vi "iv-sweep.vi"() -> ()   [LabVIEW 2010]
uses:
  <instrlib>/Keithley 24XX/Public/Data/Read (Multiple Points).vi
  <vilib>/Utility/file.llb/Write To Spreadsheet File (DBL).vi
  C/Program Files/National Instruments/LabVIEW 2016/instr.lib/Stanford Research 830/Stanford Research 830.lvlib
  C/Program Files/National Instruments/LabVIEW 2016/instr.lib/Keithley 2450/Keithley 2450.lvlib
  <instrlib>/Keithley 24XX/Keithley 24XX.lvlib
  <vilib>/Analysis/NI_AALBase.lvlib
panel:
  out "XY Graph 3":cluster{dbl[], dbl[]}(graph)={[], [3.246237e-08, 3.246237e-08]}
  in  "Parameter2 (1: X)  3":u16(ring)=2 items=["X"=1, "Y"=2, "R"=3, "Theta"=4, "Channel 1"=5, "Channel 2"=6, "Aux In 1"=7, "Aux In 2"=8, "Aux In 3"=9, "Aux In 4"=10]
  in  "Parameter (1: X) 3":u16(ring)=1 items=["X"=1, "Y"=2, "R"=3, "Theta"=4, "Channel 1"=5, "Channel 2"=6, "Aux In 1"=7, "Aux In 2"=8, "Aux In 3"=9, "Aux In 4"=10]
  in  "data number":dbl=100.0
  in  "offset(V)":dbl
  in  "Parameter2 (1: X)  2":u16(ring)=4 items=["X"=1, "Y"=2, "R"=3, "Theta"=4, "Channel 1"=5, "Channel 2"=6, "Aux In 1"=7, "Aux In 2"=8, "Aux In 3"=9, "Aux In 4"=10]
  out "PHASE":dbl=159.294
  out "LOCKIN2\n-THETA":cluster{dbl[], dbl[]}(graph)={[0.0005, 0.00045000000000000004, 0.0004, 0.00035, 0.00030000000000000003, 0.00025, 0.0002, 0.00015000000000000001, 0.0001, 5e-05, 0.0, 0.00024000000000000003, 0.00023, 0.00022, 0.00021, 0.0002, 0.00019, 0.00018, 0.00017, 0.00016, 0.00015000000000000001, 0.00014000000000000001, 0.00013000000000000002, 0.00012000000000000002, 0.00011, 0.0001, 9e-05, 8e-05, 7.000000000000001e-05, 6.000000000000001e-05, 5e-05, 4e-05, 3.0000000000000004e-05, 2e-05, 1e-05, 0.0], [159.294, 135.0, -5.628, -140.196, 157.518, -86.604, -109.212, 136.824, 42.054, -163.194, -5.196, -125.64, -38.532, -101.658, -53.202, 19.062, 69.636, -47.118, 180.0, -61.17, -36.72, 100.386, -110.046, -161.832, 112.836, 52.062, 88.626, -145.602, -128.772, -5.892, 43.392, 156.552, 66.102, -148.23, -19.77, -42.372]}
  in  "Parameter (1: X) 2":u16(ring)=3 items=["X"=1, "Y"=2, "R"=3, "Theta"=4, "Channel 1"=5, "Channel 2"=6, "Aux In 1"=7, "Aux In 2"=8, "Aux In 3"=9, "Aux In 4"=10]
  out "R Measurement 2":dbl=5.27132e-07
  out "LOVK2-r":cluster{dbl[], dbl[]}(graph)={[0.0005, 0.00045000000000000004, 0.0004, 0.00035, 0.00030000000000000003, 0.00025, 0.0002, 0.00015000000000000001, 0.0001, 5e-05, 0.0, 0.00024000000000000003, 0.00023, 0.00022, 0.00021, 0.0002, 0.00019, 0.00018, 0.00017, 0.00016, 0.00015000000000000001, 0.00014000000000000001, 0.00013000000000000002, 0.00012000000000000002, 0.00011, 0.0001, 9e-05, 8e-05, 7.000000000000001e-05, 6.000000000000001e-05, 5e-05, 4e-05, 3.0000000000000004e-05, 2e-05, 1e-05, 0.0], [5.27132e-07, 4.22822e-07, 3.52042e-07, 3.9302e-07, 4.33998e-07, 3.81844e-07, 5.01055e-07, 3.27827e-07, 2.14205e-07, 1.4715e-07, 1.84403e-07, 1.06171e-07, 5.92325e-07, 4.89879e-07, 2.83124e-07, 3.12926e-07, 2.19793e-07, 4.09784e-08, 4.65664e-08, 2.34694e-07, 3.63218e-07, 4.30273e-07, 2.58909e-07, 4.5635e-07, 7.11534e-07, 4.15372e-07, 6.98496e-07, 4.78703e-07, 5.42033e-07, 5.69973e-07, 2.6636e-07, 3.12926e-07, 2.88712e-07, 4.43311e-07, 2.62635e-07, 5.21544e-07]}
  in  "Clear Plot 2":bool
  in  "TRIGGER (1:EXTERNAL)":i32=1
  in  "REFERENCE(0:EXTERNAL)":i32
  in  "auto phase 2":bool=TRUE
  in  "manual phase 2":dbl
  in  "harm#2 2":dbl=1.0
  in  "Sine Output Amplitude (1 V) 3":dbl=0.05
  in  "Input Connection (0: Single-Ended Voltage)  2":u16(ring)=1 items=["Single-Ended Voltage", "Differential Voltage", "1 MOhm Current Gain", "100 MOhm Current Gain"]
  in  "frequency 2":dbl=50.0 format="%#_13g"
  in  "lockin-NL":refnum<visa-resource-name>="GPIB0::10::INSTR"
  out "XY Graph 2":cluster{dbl[], dbl[]}(graph)={[0.0005, 0.00045000000000000004, 0.0004, 0.00035, 0.00030000000000000003, 0.00025, 0.0002, 0.00015000000000000001, 0.0001, 5e-05, 0.0, 0.00025, 0.00024000000000000003, 0.00023, 0.00022, 0.00021, 0.0002, 0.00019, 0.00018, 0.00017, 0.00016, 0.00015000000000000001, 0.00014000000000000001, 0.00013000000000000002, 0.00012000000000000002, 0.00011, 0.0001, 9e-05, 8e-05, 7.000000000000001e-05, 6.000000000000001e-05, 5e-05, 4e-05, 3.0000000000000004e-05, 2e-05, 1e-05, 0.0], [8.888416918811881e-08, -1.8290904643564357e-07, 1.7707216663366337e-07, -2.2476362376237624e-08, 2.3799105722772277e-07, -3.8458769504950495e-08, -7.441385495049504e-09, -1.0435934356435644e-08, -1.0435934356435644e-08]}
  out "para2 Measurement":dbl=8.888416918811881e-08
  in  "auto phase":bool
  in  "manual phase":dbl
  in  "harm#2":dbl=2.0
  out "top gate leaking":dbl=-4.5445435609137164e-11
  out "top gate voltage":dbl format="%#_13g"
  in  "Compliance  Level (1uA)":dbl=3e-09
  in  "Source Mode  (0: Voltage)":u16(ring) items=["Voltage", "Current"]
  in  "top gate thickness":dbl=1.0
  in  "bottom gate thickness":dbl=1.0
  in  "pure field (T)/pure doping (F)":bool
  in  "Serial Configuration":T1={"Baud Rate"=9600, "Parity"=0, "Data Bits"=8, "Stop Bits"=10, "Flow Control"=0} {"Flow Control" items=["None", "XON/XOFF", "RTS/CTS", "XON/XOFF & RTS/CTS", "DTR/DSR", "XON/XOFF & DTR/DSR"]; "Stop Bits" items=["1.0"=10, "1.5"=15, "2.0"=20]; "Data Bits" items=["7"=7, "8"=8]; "Parity" items=["None", "Odd", "Even", "Mark", "Space"]; "Baud Rate" items=["300"=300, "600"=600, "1200"=1200, "2400"=2400, "4800"=4800, "9600"=9600, "19200"=19200]}
  in  "top gate address":refnum<visa-resource-name>="GPIB0::25::INSTR"
  out "loop run":i32=1
  in  "loop #":i32=1
  in  "Save data or not":bool
  in  "path (folder + filename)":string="C:\\Users\\User\\Data\\Jason\\07022019\\rl real other is ll\\pureE\\9v-100mv-avg-Pure E_100_new"
  in  "Clear Plot":bool
  out "XY Graph":cluster{dbl[], dbl[]}(graph)={[0.0005, 0.00045000000000000004, 0.0004, 0.00035, 0.00030000000000000003, 0.00025, 0.0002, 0.00015000000000000001, 0.0001, 5e-05, 0.0, 0.00025, 0.00024000000000000003, 0.00023, 0.00022, 0.00021, 0.0002, 0.00019, 0.00018, 0.00017, 0.00016, 0.00015000000000000001, 0.00014000000000000001, 0.00013000000000000002, 0.00012000000000000002, 0.00011, 0.0001, 9e-05, 8e-05, 7.000000000000001e-05, 6.000000000000001e-05, 5e-05, 4e-05, 3.0000000000000004e-05, 2e-05, 1e-05, 0.0], [8.142211237623763e-09, -5.9199106930693075e-09, 5.3011833564356435e-08, -6.179726722772277e-08, -1.642294698811881e-07, -1.2808030811881188e-08, -1.934349495049505e-08, 3.920102207920792e-08, 3.920102207920792e-08]}
  out "para1 Measurement":dbl=8.142211237623763e-09
  out "gate voltage":dbl format="%#_13g"
  out "gate leaking":string="3.246237E-08\n"
  in  "GATE STEP(uv)":i32=50
  in  "GATE Low Value (default 0)":dbl
  in  "GATE High Value":dbl=0.002
  in  "Function (0: Volts) 2":u16(ring) items=["Volts", "Current", "Resistance"]
  in  "Source Compaliance":dbl=3e-06
  in  "back gate address":refnum<visa-resource-name>="GPIB0::18::INSTR"
  in  "SD stabilization(S) 2":dbl=0.1 format="%#_13g"
  in  "Sine Output Amplitude (1 V) 2":dbl=2.0
  in  "LOCKIN-WAIT":dbl=0.5 format="%#_13g"
  in  "frequency":dbl=50.0 format="%#_13g"
  in  "Input Connection (0: Single-Ended Voltage)":u16(ring)=1 items=["Single-Ended Voltage", "Differential Voltage", "1 MOhm Current Gain", "100 MOhm Current Gain"]
  in  "LOCKIN address":refnum<visa-resource-name>="GPIB0::8::INSTR"
  # "Lock-in"
  # "top Gate Setting"
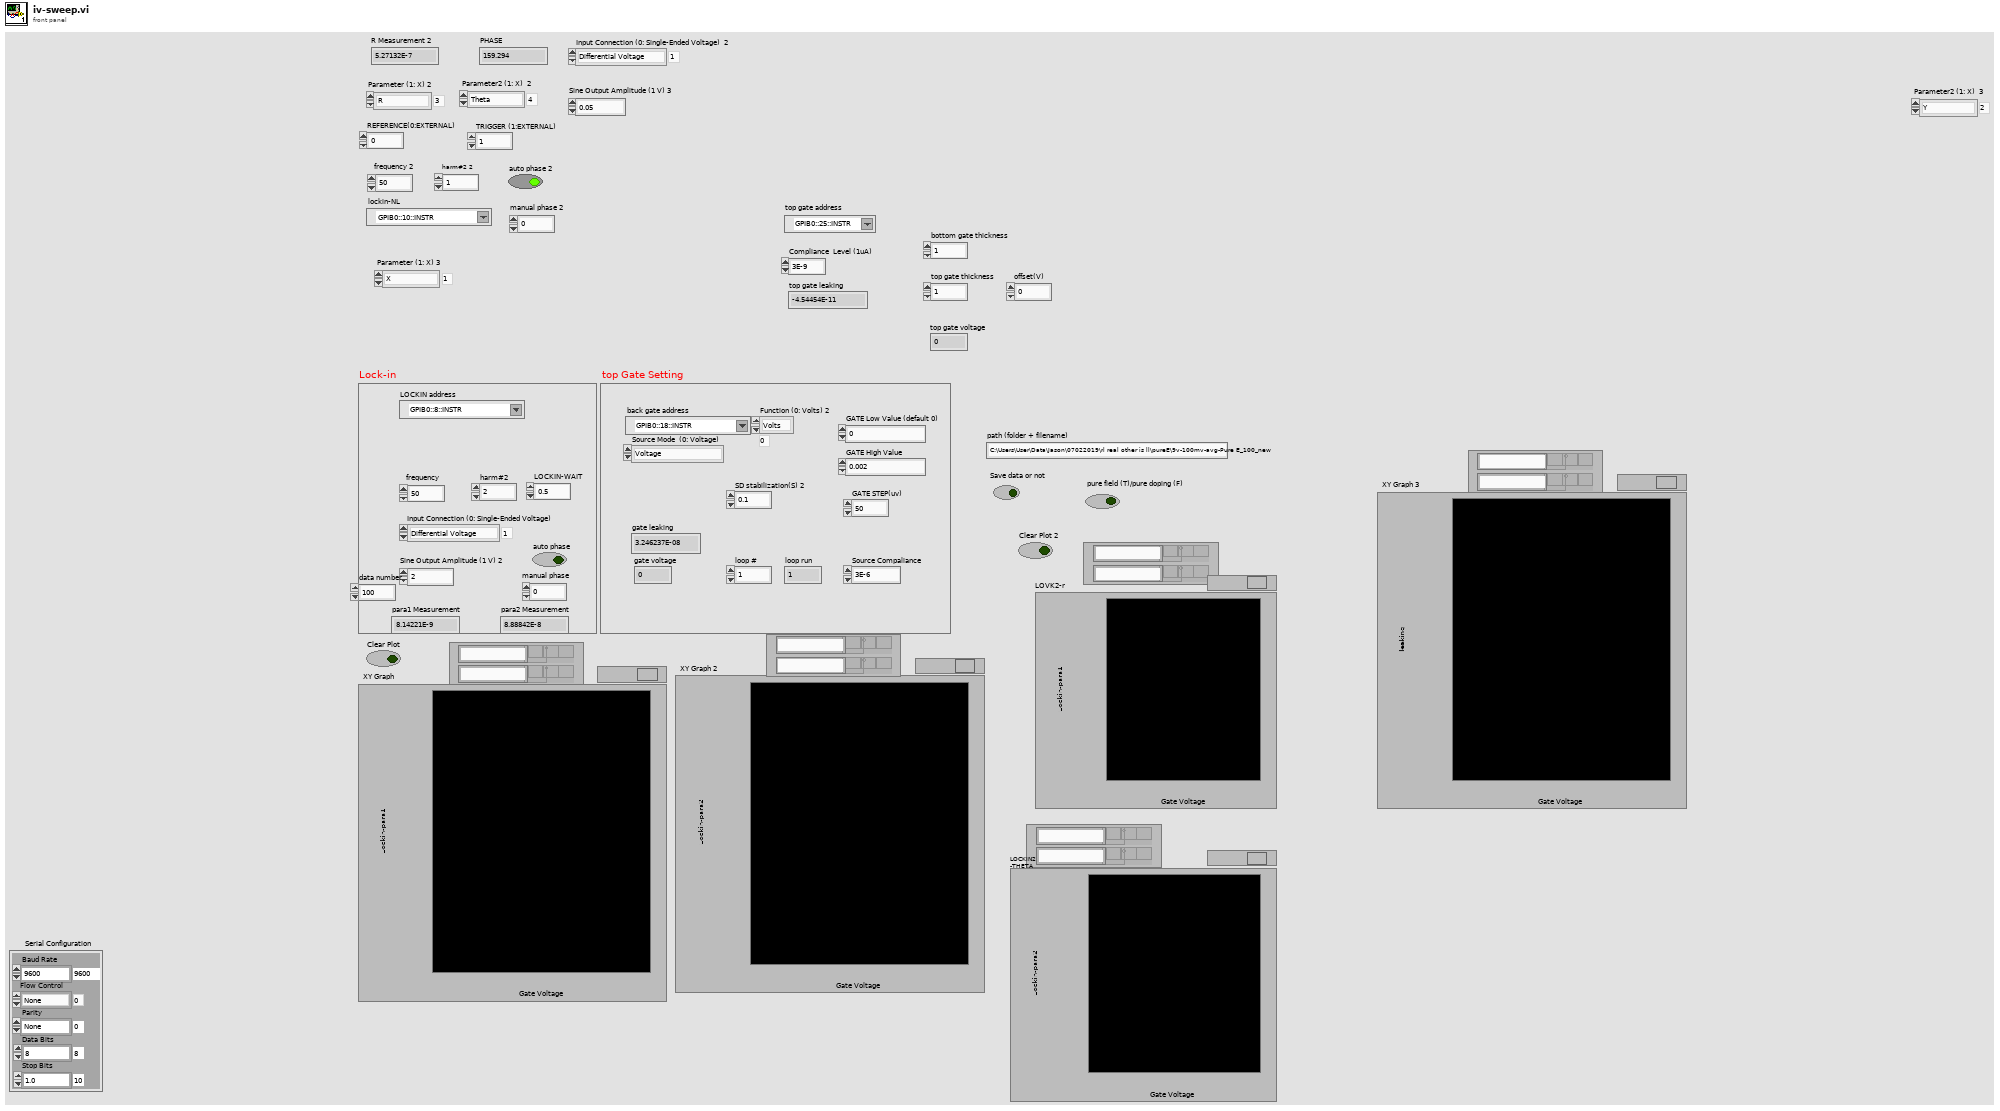
[diagram p1: front panel]
types:
  T1 = cluster{"Baud Rate":u32, "Parity":u16, "Data Bits":u16, "Stop Bits":u16, "Flow Control":u16}
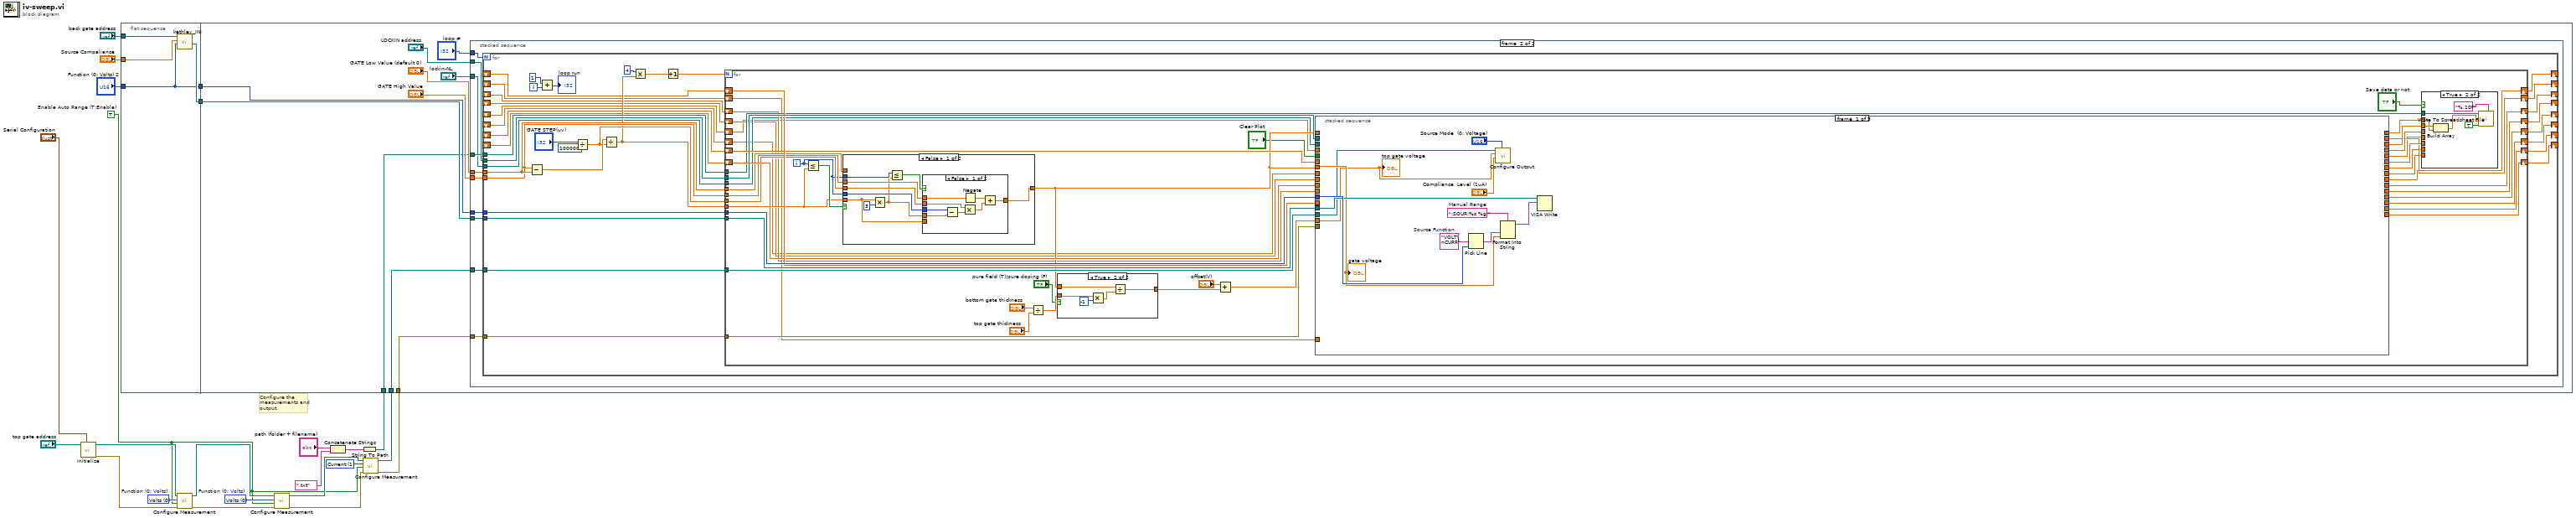
[diagram p0: block diagram]
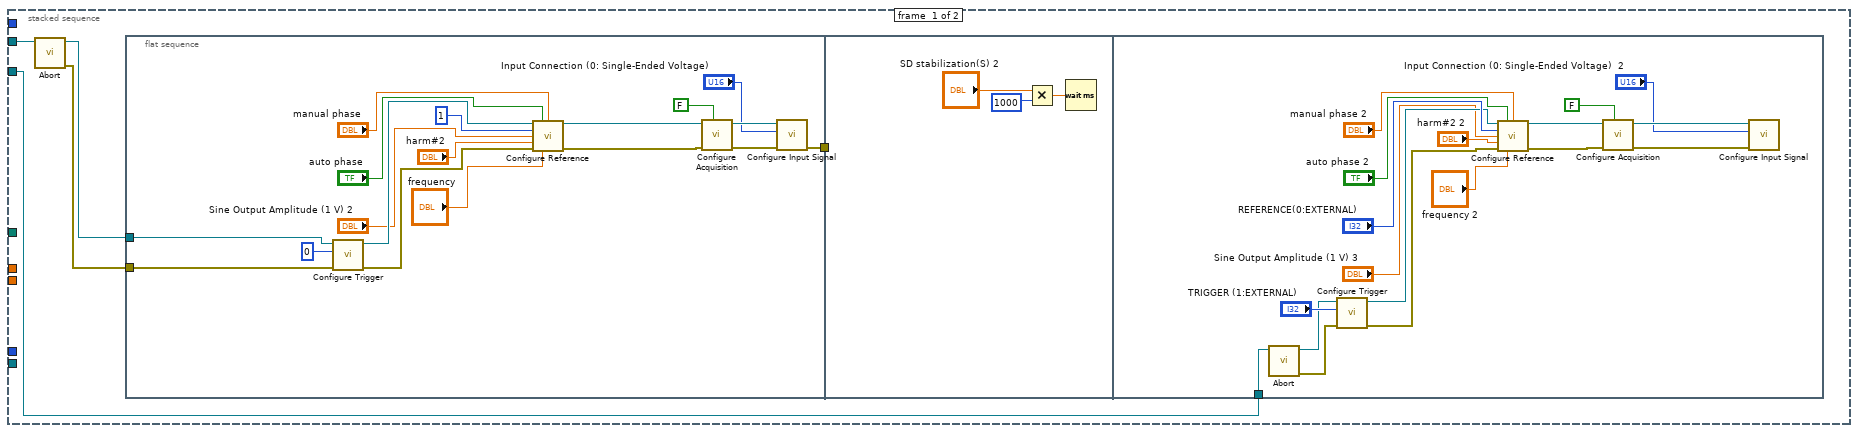
[diagram p2: hidden frame]
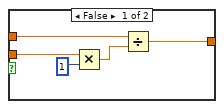
[diagram p3: hidden frame]
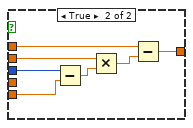
[diagram p5: hidden frame]
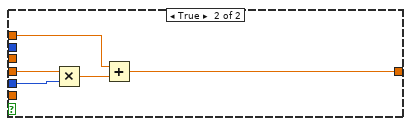
[diagram p6: hidden frame]
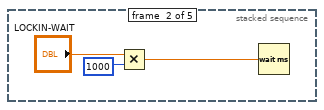
[diagram p7: hidden frame]
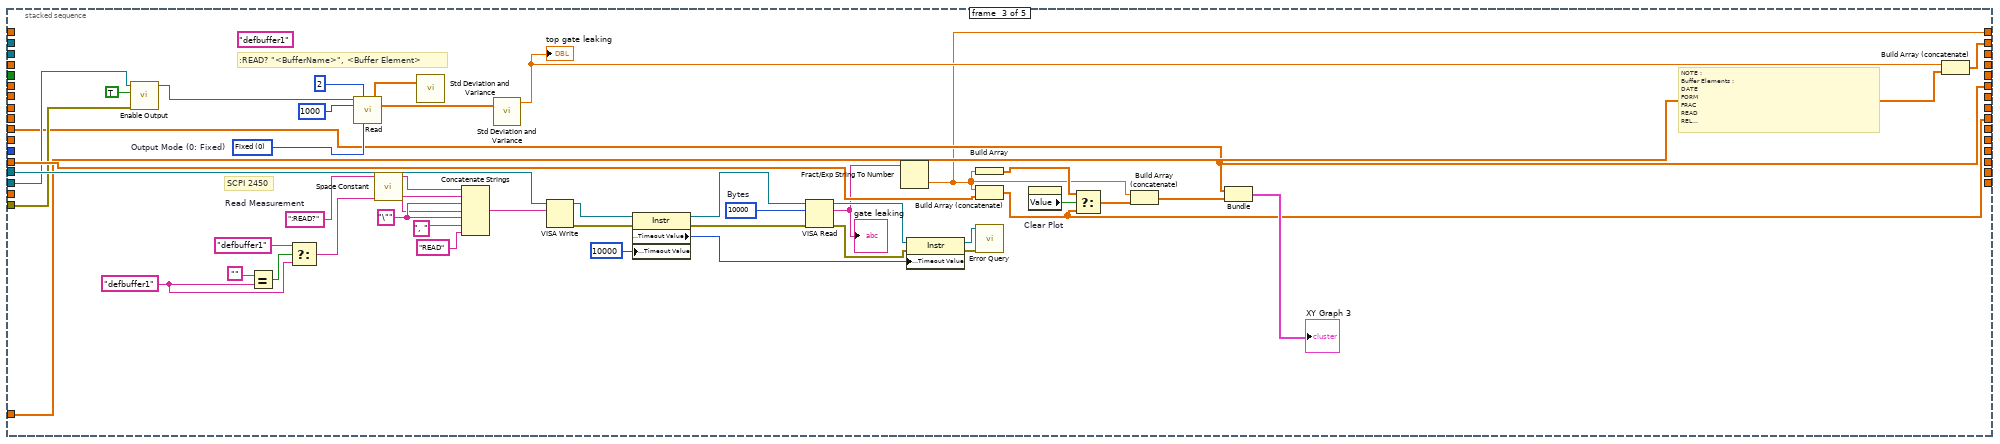
[diagram p8: hidden frame]
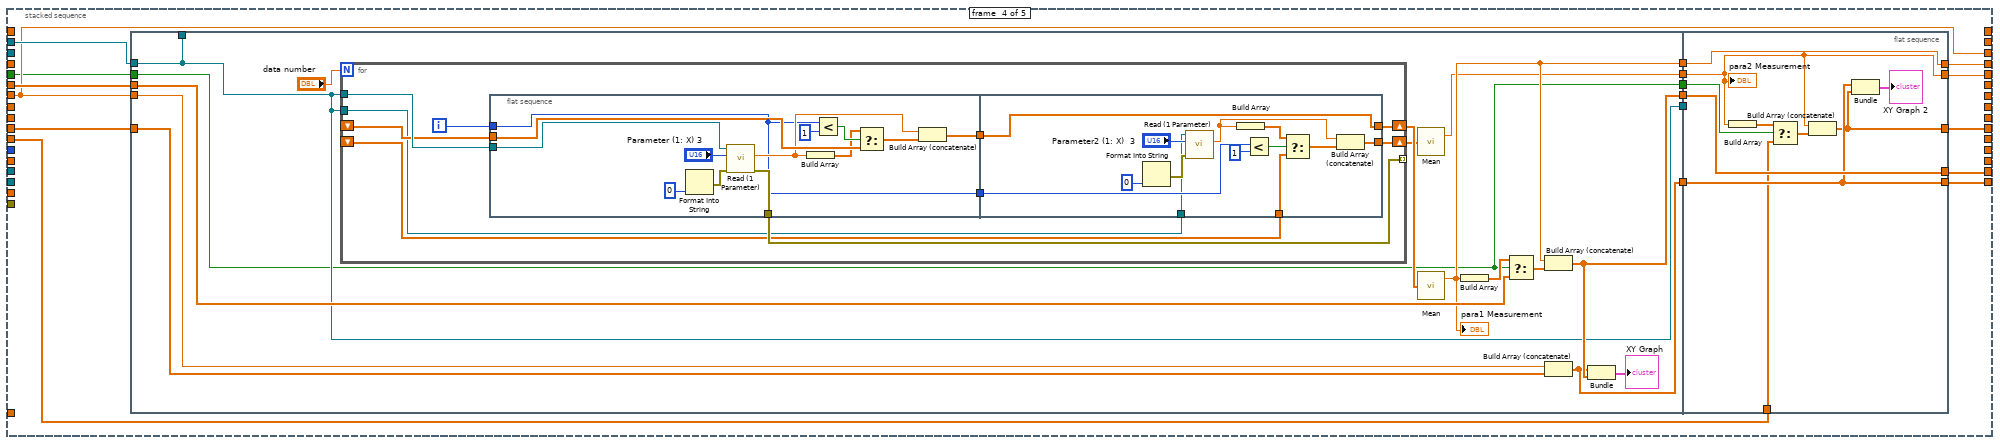
[diagram p9: hidden frame]
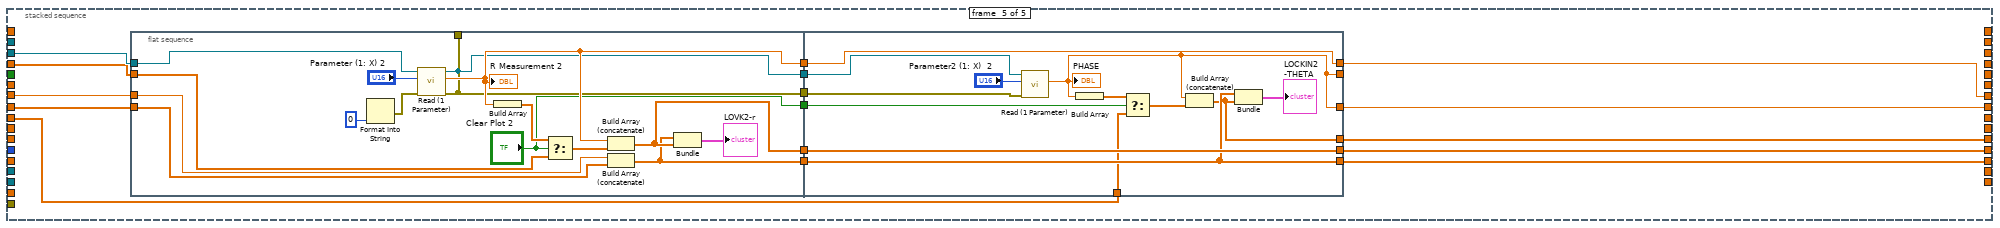
[diagram p10: hidden frame]
diagram:
  w3 = u16 1 items=["Volts", "Current", "Resistance"] ("Function (0: Volts)")
  w4 = TRUE  # Enable Auto Range (T:Enable)
  w7 = u16 0 items=["Volts", "Current", "Resistance"]  # Function (0: Volts)
  w8 = u16 0 items=["Volts", "Current", "Resistance"]  # Function (0: Volts)
  # "Configure the measurements and output."
  n1 = call <instrlib>:"Initialize.vi"("Serial Configuration"="Serial Configuration", "VISA resource name"="top gate address") -> ("error out"=w13:errorcluster, "VISA resource name out"=w14:refnum<visa-resource-name>)  [unwired: 8 in]
  n2 = flat-sequence {
    tunnel: "back gate address" -> [w27]
    tunnel: "Source Compaliance" -> [w26]
    tunnel: "Function (0: Volts) 2" -> [w24]
    tunnel: [w25] -> w20
    tunnel: [w24] -> w19
    tunnel: w20 -> [w36]
    tunnel: w19 -> [w35]
    tunnel: w15 -> [w32]
    tunnel: w2 -> [w30]
    tunnel: w1 -> [w29]
    frame #0 {
      n3 = call "kethley_INI.vi"("Function (0: Volts) in"=w24, "Source Compaliance"=w26, "VISA Refnum in"=w27) -> ("VISA resource name out"=w25:refnum<visa-resource-name>)  [unwired: 8 in]
    }
    frame #1 {
      n4 = stacked-sequence {
        tunnel: "LOCKIN address" -> [w41 w89]
        tunnel: w36 -> [_ w90]
        tunnel: w35 -> [_ w91]
        tunnel: "GATE High Value" -> [_ w87]
        tunnel: "GATE Low Value (default 0)" -> [_ w88]
        tunnel: w32 -> [_ w86]
        tunnel: "loop #" -> [_ w85]
        tunnel: w30 -> [_ w83]
        tunnel: w29 -> [_ w84]
        tunnel: "lockin-NL" -> [w38 w82]
        frame #0 {
          n5 = call "Abort.vi"("VISA resource name"=w41) -> ("error out"=w39:errorcluster, "VISA resource name out"=w40:refnum<visa-resource-name>)  [unwired: 9 in]
          n6 = flat-sequence {
            tunnel: w40 -> [w60]
            tunnel: [w45] -> w42
            tunnel: w39 -> [w44]
            tunnel: w42 -> [_]
            tunnel: w38 -> [w64]
            frame #0 {
              n7 = call "Configure Trigger.vi"("error in (no error)"=w44, "Trigger Source (0: Internal)"=0, "VISA resource name"=w60) -> ("error out"=w54:errorcluster, "VISA resource name out"=w55:refnum<visa-resource-name>)  [unwired: 7 in]
              n8 = call "Configure Reference.vi"("VISA resource name"=w55, "Auto Phase (T: Enabled)"="auto phase", "Manual Phase (0 Degree)"="manual phase", "Reference Source (1: Internal)"=1, "Sine Output Amplitude (1 V)"="Sine Output Amplitude (1 V) 2", "Detection Harmonic Number (1)"="harm#2", "error in (no error)"=w54, "Internal Reference Frequency (1000 Hz)"="frequency") -> ("VISA resource name out"=w52:refnum<visa-resource-name>, "error out"=w47:errorcluster)  [unwired: 6 in]
              n9 = call "Configure Acquisition.vi"("Continuous Storage (T: Enable)"=FALSE, "error in (no error)"=w47, "VISA resource name"=w52) -> ("error out"=w46:errorcluster, "VISA resource name out"=w50:refnum<visa-resource-name>)  [unwired: 7 in]
              n10 = call "Configure Input Signal.vi"("error in (no error)"=w46, "Input Connection (0: Single-Ended Voltage)"="Input Connection (0: Single-Ended Voltage)", "VISA resource name"=w50) -> ("error out"=w45:errorcluster)  [unwired: 7 in, 1 out]
            }
            frame #1 {
              n11 = Multiply(x="SD stabilization(S) 2", y=1000) -> (x*y=w63:dbl)
              n12 = Wait (ms)(milliseconds to wait=w63) -> ()  [unwired: 1 out]
            }
            frame #2 {
              n13 = call "Abort.vi"("VISA resource name"=w64) -> ("error out"=w65:errorcluster, "VISA resource name out"=w66:refnum<visa-resource-name>)  [unwired: 9 in]
              n14 = call "Configure Trigger.vi"("error in (no error)"=w65, "Trigger Source (0: Internal)"="TRIGGER (1:EXTERNAL)", "VISA resource name"=w66) -> ("error out"=w76:errorcluster, "VISA resource name out"=w77:refnum<visa-resource-name>)  [unwired: 7 in]
              n15 = call "Configure Reference.vi"("VISA resource name"=w77, "Auto Phase (T: Enabled)"="auto phase 2", "Manual Phase (0 Degree)"="manual phase 2", "Reference Source (1: Internal)"="REFERENCE(0:EXTERNAL)", "Sine Output Amplitude (1 V)"="Sine Output Amplitude (1 V) 3", "Detection Harmonic Number (1)"="harm#2 2", "error in (no error)"=w76, "Internal Reference Frequency (1000 Hz)"="frequency 2") -> ("VISA resource name out"=w74:refnum<visa-resource-name>, "error out"=w69:errorcluster)  [unwired: 6 in]
              n16 = call "Configure Acquisition.vi"("Continuous Storage (T: Enable)"=FALSE, "error in (no error)"=w69, "VISA resource name"=w74) -> ("error out"=w68:errorcluster, "VISA resource name out"=w72:refnum<visa-resource-name>)  [unwired: 7 in]
              n17 = call "Configure Input Signal.vi"("error in (no error)"=w68, "Input Connection (0: Single-Ended Voltage)"="Input Connection (0: Single-Ended Voltage)  2", "VISA resource name"=w72) -> ()  [unwired: 7 in, 2 out]
            }
          }
        }
        frame #1 {
          n18 = for {
            N: w85 -> [_]
            tunnel: w91 -> [w127]
            tunnel: w90 -> [w126]
            tunnel: w89 -> [w125]
            tunnel: w88 -> [w119]
            tunnel: w87 -> [w118]
            tunnel: w86 -> [w117]
            shift-right: [w113] -> _
            shift-left: _ -> [w112]
            shift-right: [w111] -> _
            shift-left: _ -> [w109]
            shift-right: [w110] -> _
            shift-left: _ -> [w108]
            tunnel: w84 -> [w104]
            tunnel: w83 -> [w103]
            shift-right: [w102] -> _
            shift-left: _ -> [w101]
            shift-right: [w100] -> _
            shift-left: _ -> [w99]
            tunnel: w82 -> [w98]
            shift-right: [w97] -> _
            shift-left: _ -> [w96]
            shift-right: [w95] -> _
            shift-left: _ -> [w94]
            shift-right: [w93] -> _
            shift-left: _ -> [w92]
            i -> [w106]
            n19 = Subtract(x=w118, y=w119) -> (x-y=w121:dbl)
            n20 = Add(x=1, y=w106) -> (x+y=→"loop run":i32)
            n21 = Divide(x="GATE STEP(uv)", y=1000000) -> (x/y=w120:dbl)
            n22 = Divide(x=w121, y=w120) -> (x/y=w116:dbl)
            n23 = Multiply(x=4, y=w116) -> (x*y=w115:dbl)
            n24 = Increment(x=w115) -> (x+1=w114:dbl)
            n25 = for {
              N: w114 -> [_]
              tunnel: w127 -> [w173]
              tunnel: w126 -> [w172]
              tunnel: w125 -> [w171]
              tunnel: w120 -> [w162]
              shift-right: [w170] -> w113
              shift-left: w112 -> [w169]
              shift-right: [w166] -> w110
              shift-left: w108 -> [w168]
              shift-right: [w165] -> w111
              shift-left: w109 -> [w167]
              tunnel: w116 -> [w160]
              tunnel: w119 -> [w163]
              tunnel: w118 -> [w161]
              tunnel: w117 -> [w155]
              tunnel: w104 -> [w149]
              tunnel: w103 -> [w148]
              shift-right: [w147] -> w102
              shift-left: w101 -> [w146]
              shift-right: [w143] -> w100
              shift-left: w99 -> [w142]
              tunnel: w98 -> [w140]
              shift-right: [w138] -> w97
              shift-left: w96 -> [w137]
              shift-right: [w136] -> w95
              shift-left: w94 -> [w135]
              shift-right: [w132] -> w93
              shift-left: w92 -> [w133]
              i -> [w159]
              n26 = Less Or Equal?(x=w159, y=w160) -> (x <= y?=w164:bool)
              n27 = case shown="False" w164 {
                tunnel: w163 -> [_ w218]
                tunnel: w159 -> [w198 w217]
                tunnel: w162 -> [w197 w216]
                tunnel: [w195 w214] -> w144
                tunnel: w161 -> [w196 _]
                tunnel: w160 -> [w191 _]
                tunnel: w159 -> [w194 _]
                frame False {
                  n28 = Multiply(x=w191, y=3) -> (x*y=w190:dbl)
                  n29 = Less Or Equal?(x=w194, y=w190) -> (x <= y?=w192:bool)
                  n30 = case shown="False" w192 {
                    tunnel: w198 -> [w206 w213]
                    tunnel: w197 -> [w204 w211]
                    tunnel: w196 -> [w200 w209]
                    tunnel: [w202 w208] -> w195
                    tunnel: w191 -> [_ w207]
                    tunnel: w190 -> [w199 _]
                    frame False {
                      n31 = Subtract(x=w206, y=w199) -> (x-y=w205:dbl)
                      n32 = Multiply(x=w204, y=w205) -> (x*y=w203:dbl)
                      n33 = Negate(x=w200) -> (-x=w201:dbl)
                      n34 = Add(x=w201, y=w203) -> (x+y=w202:dbl)
                    }
                    frame True {
                      n35 = Subtract(x=w213, y=w207) -> (x-y=w212:dbl)
                      n36 = Multiply(x=w211, y=w212) -> (x*y=w210:dbl)
                      n37 = Subtract(x=w209, y=w210) -> (x-y=w208:dbl)
                    }
                  }
                }
                frame True {
                  n38 = Multiply(x=w216, y=w217) -> (x*y=w215:dbl)
                  n39 = Add(x=w218, y=w215) -> (x+y=w214:dbl)
                }
              }
              n40 = Divide(x="bottom gate thickness", y="top gate thickness") -> (x/y=w153:dbl)
              n41 = case shown="True" "pure field (T)/pure doping (F)" {
                tunnel: w153 -> [w177 w183]
                tunnel: [w174 w181] -> w130
                tunnel: w144 -> [w175 w180]
                frame False {
                  n42 = Multiply(x=w177, y=1) -> (x*y=w176:dbl)
                  n43 = Divide(x=w175, y=w176) -> (x/y=w174:dbl)
                }
                frame True {
                  n44 = Multiply(x=w183, y=-1) -> (x*y=w179:dbl)
                  n45 = Divide(x=w180, y=w179) -> (x/y=w181:dbl)
                }
              }
              n46 = Add(x="offset(V)", y=w130) -> (x+y=w129:dbl)
              n47 = stacked-sequence {
                tunnel: w173 -> [w225 _ _ _ _]
                tunnel: w172 -> [w224 _ w255 _ _]
                tunnel: w171 -> [_ _ _ w290 _]
                tunnel: w144 -> [w223 _ _ w288 w364]
                tunnel: [_ _ w236 _ _] -> w170
                tunnel: w169 -> [_ _ w254 _ _]
                tunnel: w168 -> [_ _ _ w294 _]
                tunnel: w167 -> [_ _ w235 w291 _]
                tunnel: [_ _ _ w293 _] -> w166
                tunnel: [_ _ _ w292 _] -> w165
                tunnel: [_ _ _ w289 _] -> w158
                tunnel: [_ _ _ w288 _] -> w157
                tunnel: [_ _ w235 _ _] -> w156
                tunnel: w129 -> [w220 _ _ _ _]
                tunnel: w149 -> [_ _ w245 _ _]
                tunnel: w148 -> [w219 _ w244 _ _]
                tunnel: [_ _ w243 _ _] -> w147
                tunnel: w146 -> [_ _ w242 _ _]
                tunnel: [_ _ w233 _ _] -> w145
                tunnel: w144 -> [_ _ _ _ _]
                tunnel: [_ _ _ w282 _] -> w143
                tunnel: w142 -> [_ _ _ w279 _]
                tunnel: [_ _ _ w281 _] -> w141
                tunnel: w140 -> [_ _ _ _ w365]
                tunnel: [_ _ _ _ w363] -> w139
                tunnel: [_ _ _ _ w362] -> w138
                tunnel: w137 -> [_ _ _ _ w361]
                tunnel: [_ _ _ _ w360] -> w136
                tunnel: w135 -> [_ _ _ _ w359]
                tunnel: [_ _ _ _ w358] -> w134
                tunnel: w133 -> [_ _ _ _ w357]
                tunnel: [_ _ _ _ w356] -> w132
                tunnel: "Clear Plot" -> [_ _ _ w278 _]
                frame #0 {
                  w227 = "VOLT\nCURR"  # Source Function
                  w228 = ":SOUR:%s %g;"  # Manual Range
                  n48 = Pick Line(multi-line string=w227, line index=w225) -> (output string=w226:string)  [unwired: 1 out]
                  n49 = call <instrlib>:"Configure Output.vi"("Source Mode  (0: Voltage)"="Source Mode  (0: Voltage)", "Compliance  Level (0.1)"="Compliance  Level (1uA)", "Output Level (0)"=w220, "VISA resource name"=w219) -> ()  [unwired: 6 in, 2 out]
                  n50 = Format Into String(format string=w228, w226, w223) -> (resulting string=w229:string)  [unwired: 2 in, 1 out]
                  n51 = VISA Write(VISA resource name=w224, write buffer=w229) -> ()  [unwired: 1 in, 3 out]
                  "gate voltage" <- w223
                  "top gate voltage" <- w220
                }
                frame #1 {
                  n52 = Multiply(x="LOCKIN-WAIT", y=1000) -> (x*y=w232:dbl)
                  n53 = Wait (ms)(milliseconds to wait=w232) -> ()  [unwired: 1 out]
                }
                frame #2 {
                  w250 = u16 0 items=["Fixed", "Sweep", "List"]  # Output Mode (0: Fixed)
                  w266 = "defbuffer1" ("Buffer Name (defbuffer1) 2")
                  (unwired) "defbuffer1" ("t")
                  w264 = "\""
                  w261 = ":READ?"  # Read Measurement
                  w270 = u32 10000  # Bytes
                  # "NOTE :\nBuffer Elements :\nDATE\nFORM\nFRAC\nREAD\nREL\nSEC\nSOUR\nSOURFORM\nSOURSTAT\nSOURUNIT\nSTAT\nTIME\nTsT\nUNIT"
                  # ":READ? \"<BufferName>\", <Buffer Element>"
                  # "SCPI 2450"
                  n54 = call <instrlib>:"Enable Output.vi"("error in (no error)"=w245, "Enable Output (T: Enable)"=TRUE, "VISA resource name"=w244) -> ("VISA resource name out"=w246:refnum<visa-resource-name>)  [unwired: 7 in, 1 out]
                  n55 = Equal?(x="", y=w266) -> (x = y?=w267:bool)
                  n56 = Select(t="defbuffer1", s=w267, f=w266) -> (s? t:f=w263:string)
                  n57 = call-poly <instrlib>:"Read.vi"("VISA resource name"=w246, "Sample Count (1)"=u32 2 ("Number of Samples"), "Timeout (10000 ms)"=1000, "Output Mode (0: Fixed)"=w250) -> ("Voltage"=w248:sgl[], "Current"=w249:sgl[])  [unwired: 5 in, 5 out]
                  n58 = call <vilib>:"Space Constant.vi"() -> ("String"=w262:string)
                  n59 = call <vilib>:"Std Deviation and Variance.vi"("X"=w248) -> ()  [unwired: 1 in, 3 out]
                  n60 = Concatenate Strings(w261, w262, w264, w263, w264, ", " ("string"), "READ" ("Buffer Elements 2")) -> (w277:string)
                  n61 = call <vilib>:"Std Deviation and Variance.vi"("X"=w249) -> ("mean"=w234:dbl)  [unwired: 1 in, 2 out]
                  "top gate leaking" <- w234
                  n62 = VISA Write(VISA resource name=w255, write buffer=w277) -> (VISA resource name out=w269:refnum<visa-resource-name>, error out=w276:errorcluster)  [unwired: 1 in, 1 out]
                  n63 = property class="Instr"(reference=w269, error in=w276, "General Settings:Timeout Value"=10000 ("Timeout (10000 ms) 2")) -> (reference out=w275:refnum<visa-resource-name>, error out=w274:errorcluster, "General Settings:Timeout Value"=w271:u32)
                  n64 = VISA Read(VISA resource name=w275, byte count=w270, error in (no error)=w274) -> (VISA resource name out=w273:refnum<visa-resource-name>, read buffer=w253:string, error out=w272:errorcluster)  [unwired: 1 out]
                  "gate leaking" <- w253
                  n65 = Fract/Exp String To Number(string=w253) -> (number=w233:dbl)  [unwired: 3 in, 1 out]
                  n66 = property class="Instr"(reference=w273, error in=w272, "General Settings:Timeout Value"=w271) -> (reference out=w259:refnum<visa-resource-name>, error out=w258:errorcluster)
                  n67 = Build Array(w233) -> (w240:dbl[])
                  n68 = Build Array (concatenate)(w233, w254) -> (w236:dbl[])
                  n69 = call "Error Query.vi"("error in (no error)"=w258, "VISA resource name"=w259) -> ()  [unwired: 10 out]
                  n70 = property on="Clear Plot" class="Bool (strict)"() -> ("Value"=w237:bool)  [unwired: 2 in, 2 out]
                  n71 = Select(t=w240, s=w237, f=w236) -> (s? t:f=w241:dbl[])
                  n72 = Build Array (concatenate)(w233, w241) -> (w238:dbl[])
                  n73 = Bundle(w235, w238) -> (→"XY Graph 3":cluster{dbl[], dbl[]})  [unwired: 1 in]
                  n74 = Build Array (concatenate)(w234, w242) -> (w243:dbl[])
                }
                frame #3 {
                  n75 = flat-sequence {
                    tunnel: w294 -> [w306]
                    tunnel: w291 -> [w303]
                    tunnel: w290 -> [w300]
                    tunnel: w288 -> [w302]
                    tunnel: [w300] -> _
                    tunnel: [w305] -> w287
                    tunnel: [w304] -> w286
                    tunnel: [w298] -> w285
                    tunnel: [w300] -> w284
                    tunnel: [w295] -> w283
                    tunnel: [w296] -> w280
                    tunnel: w278 -> [w295]
                    tunnel: [w354] -> w289
                    tunnel: [w351] -> w292
                    tunnel: [w355] -> w293
                    tunnel: w287 -> [w355]
                    tunnel: w286 -> [w351]
                    tunnel: w285 -> [w354]
                    tunnel: w284 -> [_]
                    tunnel: w283 -> [w352]
                    tunnel: [w349] -> w282
                    tunnel: [w347] -> w281
                    tunnel: w280 -> [w347]
                    tunnel: w279 -> [w346]
                    frame #0 {
                      n76 = for {
                        N: "data number" -> [_]
                        tunnel: w300 -> [w319]
                        shift-right: [w318] -> w299
                        shift-left: _ -> [w315]
                        tunnel: [w317] -> _ mode=indexing
                        tunnel: w300 -> [w312]
                        shift-right: [w311] -> w297
                        shift-left: _ -> [w310]
                        i -> [w316]
                        n77 = flat-sequence {
                          tunnel: w319 -> [w331]
                          tunnel: [w327] -> w317
                          tunnel: w316 -> [w320]
                          tunnel: w315 -> [w324]
                          tunnel: [w328] -> w314
                          tunnel: [w320] -> w313
                          tunnel: [w345] -> w318
                          tunnel: w314 -> [w345]
                          tunnel: w313 -> [w336]
                          tunnel: w312 -> [w335]
                          tunnel: [w334] -> w311
                          tunnel: w310 -> [w333]
                          frame #0 {
                            n78 = Format Into String(0) -> (error out=w329:errorcluster)  [unwired: 3 in, 1 out]
                            n79 = call "Read (1 Parameter).vi"("error in (no error)"=w329, "Parameter (1: X)"="Parameter (1: X) 3", "VISA resource name"=w331) -> ("error out"=w327:errorcluster, "Measurement"=w322:dbl)  [unwired: 6 in, 1 out]
                            n80 = Build Array(w322) -> (w321:dbl[])
                            n81 = Less?(x=w320, y=1) -> (x < y?=w325:bool)
                            n82 = Select(t=w321, s=w325, f=w324) -> (s? t:f=w323:dbl[])
                            n83 = Build Array (concatenate)(w322, w323) -> (w328:dbl[])
                          }
                          frame #1 {
                            n84 = Format Into String(0) -> (error out=w343:errorcluster)  [unwired: 3 in, 1 out]
                            n85 = call "Read (1 Parameter).vi"("error in (no error)"=w343, "Parameter (1: X)"="Parameter2 (1: X)  3", "VISA resource name"=w335) -> ("Measurement"=w338:dbl)  [unwired: 6 in, 2 out]
                            n86 = Build Array(w338) -> (w339:dbl[])
                            n87 = Less?(x=w336, y=1) -> (x < y?=w340:bool)
                            n88 = Select(t=w339, s=w340, f=w333) -> (s? t:f=w337:dbl[])
                            n89 = Build Array (concatenate)(w338, w337) -> (w334:dbl[])
                          }
                        }
                      }
                      n90 = call <vilib>:"Mean.vi"("X"=w297) -> ("mean"=w296:dbl)  [unwired: 1 out]
                      n91 = call <vilib>:"Mean.vi"("X"=w299) -> ("mean"=w298:dbl)  [unwired: 1 out]
                      "para1 Measurement" <- w298
                      n92 = Build Array(w298) -> (w308:dbl[])
                      n93 = Select(t=w308, s=w295, f=w306) -> (s? t:f=w309:dbl[])
                      n94 = Build Array (concatenate)(w298, w309) -> (w305:dbl[])
                      n95 = Build Array (concatenate)(w302, w303) -> (w304:dbl[])
                      n96 = Bundle(w304, w305) -> (→"XY Graph":cluster{dbl[], dbl[]})  [unwired: 1 in]
                    }
                    frame #1 {
                      n97 = Build Array(w347) -> (w353:dbl[])
                      n98 = Select(t=w353, s=w352, f=w346) -> (s? t:f=w350:dbl[])
                      n99 = Build Array (concatenate)(w347, w350) -> (w349:dbl[])
                      n100 = Bundle(w351, w349) -> (→"XY Graph 2":cluster{dbl[], dbl[]})  [unwired: 1 in]
                      "para2 Measurement" <- w347
                    }
                  }
                }
                frame #4 {
                  n101 = flat-sequence {
                    tunnel: w365 -> [w380]
                    tunnel: w364 -> [w378]
                    tunnel: [w376] -> _
                    tunnel: [w377] -> _
                    tunnel: [w382] -> w371
                    tunnel: [w381] -> w370
                    tunnel: [w379] -> w369
                    tunnel: [w377] -> w368
                    tunnel: [w376] -> w367
                    tunnel: ["Clear Plot 2"] -> w366
                    tunnel: w359 -> [w374]
                    tunnel: w357 -> [w372]
                    tunnel: [w399] -> w358
                    tunnel: [w393] -> w356
                    tunnel: [w400] -> w360
                    tunnel: w371 -> [w400]
                    tunnel: w370 -> [w393]
                    tunnel: w369 -> [w399]
                    tunnel: w368 -> [w397]
                    tunnel: w367 -> [w396]
                    tunnel: w366 -> [w394]
                    tunnel: [w391] -> w362
                    tunnel: [w389] -> _
                    tunnel: [w389] -> w363
                    tunnel: w361 -> [w388]
                    frame #0 {
                      n102 = Format Into String(0) -> (error out=w387:errorcluster)  [unwired: 3 in, 1 out]
                      n103 = call "Read (1 Parameter).vi"("error in (no error)"=w387, "Parameter (1: X)"="Parameter (1: X) 2", "VISA resource name"=w380) -> ("error out"=w377:errorcluster, "Measurement"=w379:dbl, "VISA resource name out"=w376:refnum<visa-resource-name>)  [unwired: 6 in]
                      "R Measurement 2" <- w379
                      n104 = Build Array(w379) -> (w385:dbl[])
                      n105 = Select(t=w385, s="Clear Plot 2", f=w374) -> (s? t:f=w373:dbl[])
                      n106 = Build Array (concatenate)(w379, w373) -> (w382:dbl[])
                      n107 = Build Array (concatenate)(w378, w372) -> (w381:dbl[])
                      n108 = Bundle(w381, w382) -> (→"LOVK2-r":cluster{dbl[], dbl[]})  [unwired: 1 in]
                    }
                    frame #1 {
                      n109 = call "Read (1 Parameter).vi"("error in (no error)"=w397, "Parameter (1: X)"="Parameter2 (1: X)  2", "VISA resource name"=w396) -> ("Measurement"=w389:dbl)  [unwired: 6 in, 2 out]
                      "PHASE" <- w389
                      n110 = Build Array(w389) -> (w395:dbl[])
                      n111 = Select(t=w395, s=w394, f=w388) -> (s? t:f=w392:dbl[])
                      n112 = Build Array (concatenate)(w389, w392) -> (w391:dbl[])
                      n113 = Bundle(w393, w391) -> (→"LOCKIN2\n-THETA":cluster{dbl[], dbl[]})  [unwired: 1 in]
                    }
                  }
                }
              }
              n114 = case shown="True" "Save data or not" {
                tunnel: w158 -> [_ _]
                tunnel: w157 -> [_ w189]
                tunnel: w156 -> [_ _]
                tunnel: w155 -> [_ w187]
                tunnel: w145 -> [_ w184]
                tunnel: w141 -> [_ _]
                tunnel: w139 -> [_ _]
                tunnel: w134 -> [_ _]
                frame False {
                }
                frame True {
                  n115 = Build Array(w189, w184) -> (w188:dbl[])
                  n116 = call-poly <vilib>:"Write To Spreadsheet File.vi"("format (%.3f)"="%.10f", "append to file? (new file:F)"=TRUE, "1D data"=w188, "file path (dialog if empty)"=w187) -> ()  [unwired: 4 in, 1 out]
                }
              }
            }
          }
        }
      }
    }
  }
  n117 = call <instrlib>:"Configure Measurement.vi"("error in (no error)"=w13, "Enable Auto Range (T:Enable)"=w4, "Function (0: Volts)"=w8, "VISA resource name"=w14) -> ("error out"=w12:errorcluster, "VISA resource name out"=w11:refnum<visa-resource-name>)  [unwired: 6 in]
  n118 = call <instrlib>:"Configure Measurement.vi"("error in (no error)"=w12, "Enable Auto Range (T:Enable)"=w4, "Function (0: Volts)"=w7, "VISA resource name"=w11) -> ("error out"=w5:errorcluster, "VISA resource name out"=w6:refnum<visa-resource-name>)  [unwired: 6 in]
  n119 = Concatenate Strings("path (folder + filename)", ".txt") -> (w16:string)
  n120 = String To Path(string=w16) -> (path=w15:path)
  n121 = call <instrlib>:"Configure Measurement.vi"("error in (no error)"=w5, "Enable Auto Range (T:Enable)"=w4, "Function (0: Volts)"=w3, "VISA resource name"=w6) -> ("error out"=w1:errorcluster, "VISA resource name out"=w2:refnum<visa-resource-name>)  [unwired: 6 in]
